vi "ArrayToExcel.vi"() -> ()   [LabVIEW 2020]
uses:
  <vilib>/Analysis/NI_AALBase.lvlib
panel:
  out "tabla":string[][](array[string])
  out "Waveform Graph":dbl[][](graph)
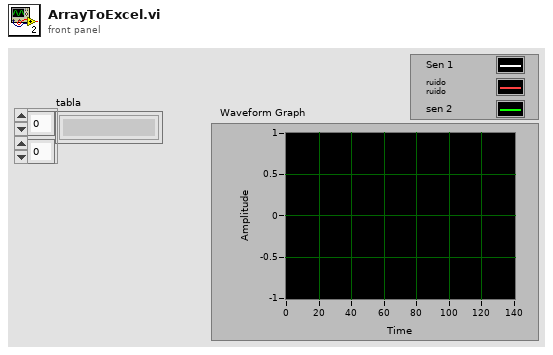
[diagram p1: front panel]
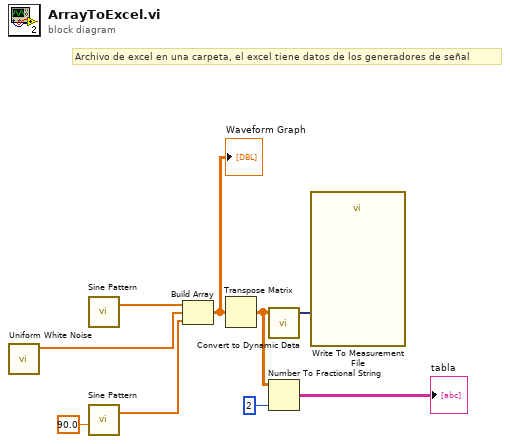
[diagram p0: block diagram]
diagram:
  # "Archivo de excel en una carpeta, el excel tiene datos de los generadores de señal"
  n1 = call <vilib>:"Uniform White Noise.vi"() -> ("uniform white noise"=w7:dbl[])  [unwired: 10 in, 1 out]
  n2 = call <vilib>:"Sine Pattern.vi"() -> ("Sinusoidal Pattern"=w8:dbl[])  [unwired: 4 in, 1 out]
  n3 = call <vilib>:"Sine Pattern.vi"("phase(degrees)"=90.0) -> ("Sinusoidal Pattern"=w6:dbl[])  [unwired: 3 in, 1 out]
  n4 = Build Array(w8, w7, w6) -> (w5:dbl[][])
  "Waveform Graph" <- w5
  n5 = Transpose Matrix(1:w5) -> (0:w4:dbl[][])
  n6 = call "Convert to Dynamic Data"("2D Array"=w4) -> ("Dynamic Data Type"=w3:dynamicdata)  [unwired: 3 in]
  n7 = Number To Fractional String(number=w4, precision (6)=i16 2) -> (F-format string=→"tabla":string[][])  [unwired: 2 in]
  n8 = call "Write To Measurement File"("Signals"=w3) -> ()  [unwired: 16 in, 3 out]
